vi "Obtain VISA Lock Ref.vi"(8 "error in (no error)":errorcluster, 11 "VISA session in":refnum<visa-resource-name>) -> (0 "error out":errorcluster, 3 "VISA session out":refnum<visa-resource-name>)   [LabVIEW 2016, in "MB_VISA_Lock.lvlib"]
doc: "Obtains the reference for the VISA resource lock. This reference is stored in the UserData property of the output VISA session. This VI should be called just after the VISA session is opened."
uses:
  MB_VISA_Lock.lvlib
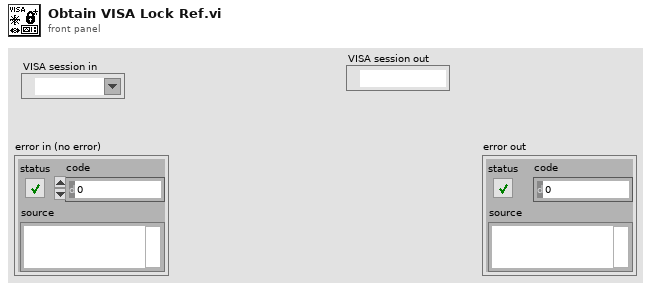
[diagram p1: front panel]
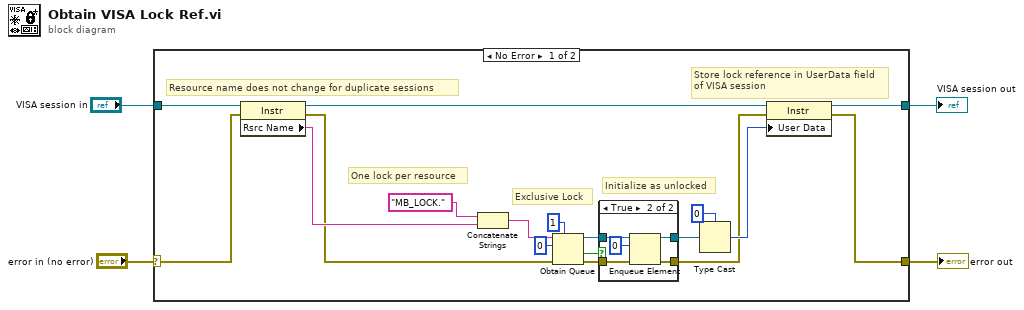
[diagram p0: block diagram]
diagram:
  n1 = case shown="No Error" "error in (no error)" {
    selector: "error in (no error)" -> [w21 w31]
    tunnel: [w20 w31] -> w4
    tunnel: "VISA session in" -> [w22 w30]
    tunnel: [w19 w30] -> w1
    frame No Error {
      # "Resource name does not change for duplicate sessions"
      # "One lock per resource"
      # "Initialize as unlocked"
      # "Store lock reference in UserData field\nof VISA session"
      # "Exclusive Lock"
      n2 = property class="Instr"(reference=w22, error in=w21) -> (reference out=w7:refnum<visa-resource-name>, error out=w10:errorcluster, "Rsrc Name"=w11:string)
      n3 = Concatenate Strings("MB_LOCK.", w11) -> (w12:string)
      n4 = Obtain Queue(max queue size (-1, unlimited)=1, name (unnamed)=w12, element data type=0, error in (no error)=w10) -> (queue out=w16:refnum<queue>, created new?=w14:bool, error out=w15:errorcluster)  [unwired: 1 in]
      n5 = case shown="True" w14 {
        tunnel: w16 -> [w24 w28]
        tunnel: w15 -> [w23 w27]
        tunnel: [w24 w26] -> w9
        tunnel: [w23 w25] -> w5
        frame False {
        }
        frame True {
          n6 = Enqueue Element(queue=w28, element=0, error in (no error)=w27) -> (queue out=w26:refnum<queue>, error out=w25:errorcluster)  [unwired: 1 in, 1 out]
        }
      }
      n7 = Type Cast(type=u32 0, x=w9) -> (*(type *) &x=w6:u32)
      n8 = property class="Instr"(reference=w7, error in=w5, "User Data"=w6) -> (reference out=w19:refnum<visa-resource-name>, error out=w20:errorcluster)
    }
    frame Error {
    }
  }
  "error out" <- w4
  "VISA session out" <- w1
